vi "Receiver.Test.vi"() -> ()   [LabVIEW 2016]
uses:
  C:/Program Files (x86)/National Instruments/LabVIEW 2016/vi.lib/Distrio/LabbitMQ/RabbitMQ.Client.dll
  Program Files (x86)/National Instruments/LabVIEW 2016/vi.lib/Distrio/LabbitMQ/RabbitMQ.Client.dll
  <vilib>/Distrio/LabbitMQ/Queue/Queue.lvclass
  <vilib>/Distrio/LabbitMQ/Connection/Connection.lvclass
panel:
  out "ReplyTo":string
  in  "queue \nname":string
  in  "exchange name":u16(ring) items=["requests", "alerts"]
  out "error out":errorcluster
  out "consumer: received message":string
  in  "binding key":string[](array[string])=["broadcast.#"]
  in  "error (in)":errorcluster
  in  "host name":string="higgsino.physics.ucsb.edu"
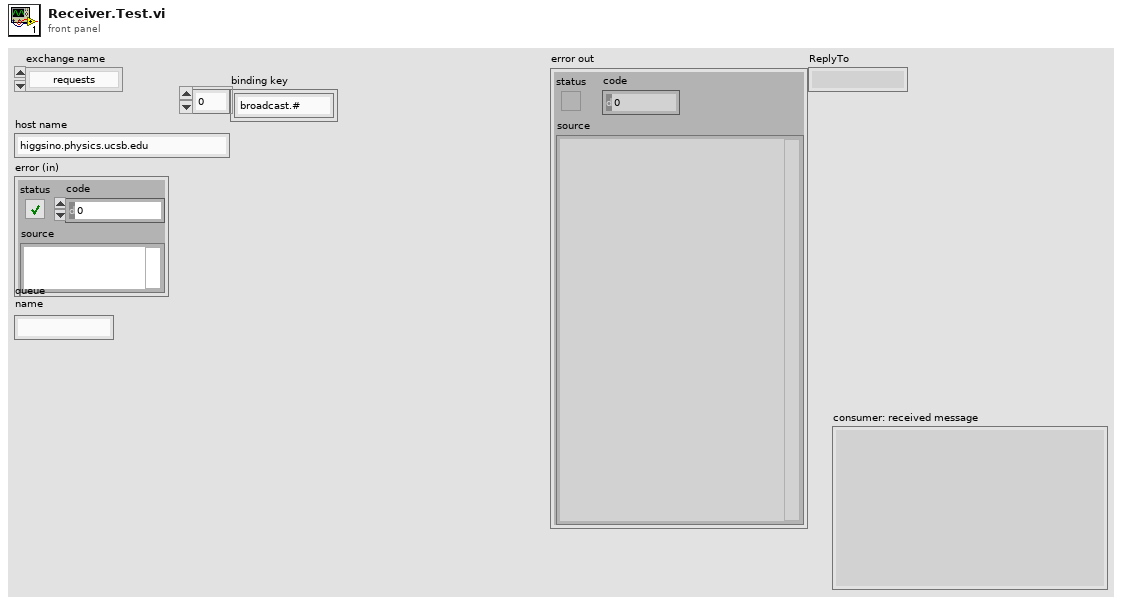
[diagram p1: front panel]
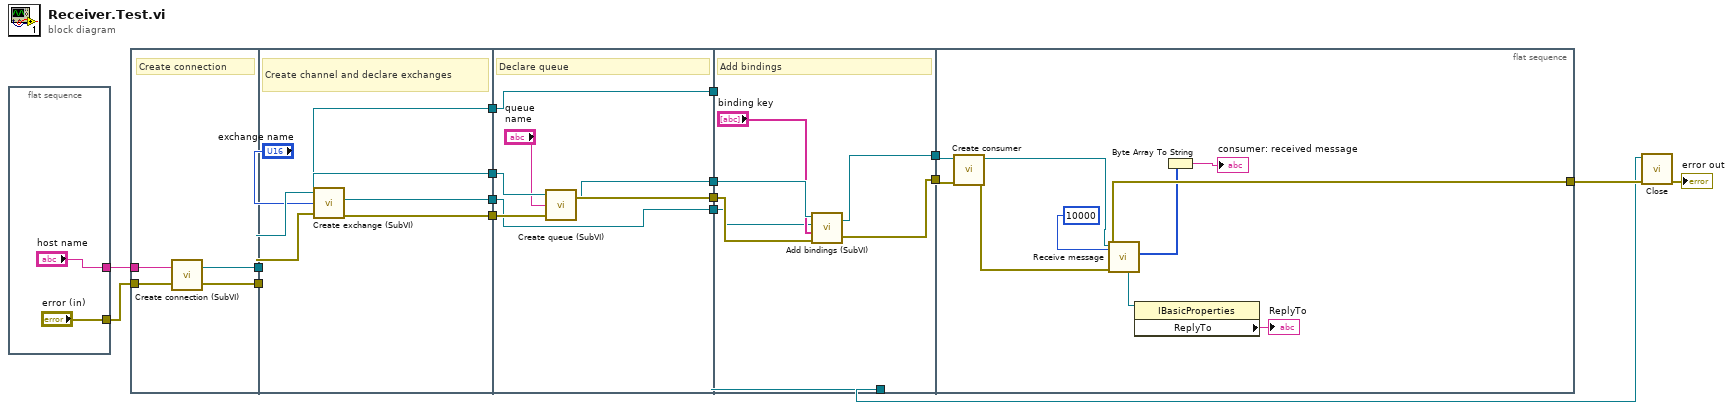
[diagram p0: block diagram]
diagram:
  n1 = flat-sequence {
    tunnel: ["error (in)"] -> w17
    tunnel: ["host name"] -> w16
    frame #0 {
    }
  }
  n2 = flat-sequence {
    tunnel: [w21] -> w15
    tunnel: [w20] -> w14
    tunnel: w16 -> [w23]
    tunnel: w17 -> [w22]
    tunnel: w15 -> [w30]
    tunnel: w14 -> [w29]
    tunnel: [w27] -> w7
    tunnel: [w26] -> w6
    tunnel: [w25] -> w5
    tunnel: [w24] -> w2
    tunnel: [w37] -> w13
    tunnel: [w36] -> w12
    tunnel: w7 -> [w35]
    tunnel: w6 -> [w34]
    tunnel: w5 -> [w33]
    tunnel: [w33] -> w4
    tunnel: [w32] -> w3
    tunnel: w2 -> [w32]
    tunnel: w13 -> [w40]
    tunnel: w12 -> [w44]
    tunnel: [w42] -> w11
    tunnel: [w41] -> w10
    tunnel: w4 -> [w39]
    tunnel: w3 -> [w38]
    tunnel: [w38] -> w1
    tunnel: w11 -> [w53]
    tunnel: w10 -> [w52]
    tunnel: [w51] -> w9
    frame #0 {
      # "Create connection"
      n3 = call "Create connection (SubVI).vi"("error in (no error)"=w22, "host name"=w23) -> ("error out"=w20:errorcluster, "Connection out"=w21:refnum<class "Connection.lvclass">)
    }
    frame #1 {
      # "Create channel and declare exchanges"
      n4 = call "Create exchange (SubVI).vi"("Connection in"=w30, "exchange name"="exchange name", "error in (no error)"=w29) -> ("Connection out"=w24:refnum<class "Connection.lvclass">, "Exchange.lvclass"=w25:refnum<class "Exchange.lvclass">, "Channel out"=w27:refnum<class "Channel.lvclass">, "error out"=w26:errorcluster)
    }
    frame #2 {
      # "Declare queue"
      n5 = call "Create queue (SubVI).vi"("error in (no error)"=w34, "queue"="queue \nname", "Channel in"=w35) -> ("error out"=w37:errorcluster, "Queue out"=w36:refnum<class "Queue.lvclass">)
    }
    frame #3 {
      # "Add bindings"
      n6 = call "Add bindings (SubVI).vi"("error in (no error)"=w40, "binding key"="binding key", "Exchange.lvclass"=w39, "Queue in"=w44) -> ("error out"=w41:errorcluster, "Queue out"=w42:refnum<class "Queue.lvclass">)
    }
    frame #4 {
      n7 = call <vilib>:"Create consumer.vi"("error in (no error)"=w52, "Queue in"=w53) -> ("error out"=w50:errorcluster, "Queue out"=w54:refnum<class "Queue.lvclass">)  [unwired: 8 in]
      n8 = call <vilib>:"Receive message.vi"("millisecondsTimeout"=10000, "error in (no error)"=w50, "Consumer in"=w54) -> ("error out"=w51:errorcluster, "message body"=w48:u8[], "MessageProperties"=w46:refnum<k24>)  [unwired: 3 in, 3 out]
      n9 = property class="IBasicProperties"(reference=w46) -> ("ReplyTo"=→"ReplyTo":string)  [unwired: 1 in, 2 out]
      n10 = Byte Array To String(unsigned byte array=w48) -> (string=→"consumer: received message":string)
    }
  }
  n11 = call <vilib>:"Close.vi"("error in (no error)"=w9, "Connection in"=w1) -> ("error out"=→"error out":errorcluster)  [unwired: 8 in, 1 out]
